vi "Producer consumer.vi"() -> ()   [LabVIEW 2021]
panel:
  in  "stop":bool
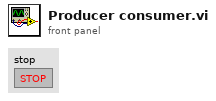
[diagram p1: front panel]
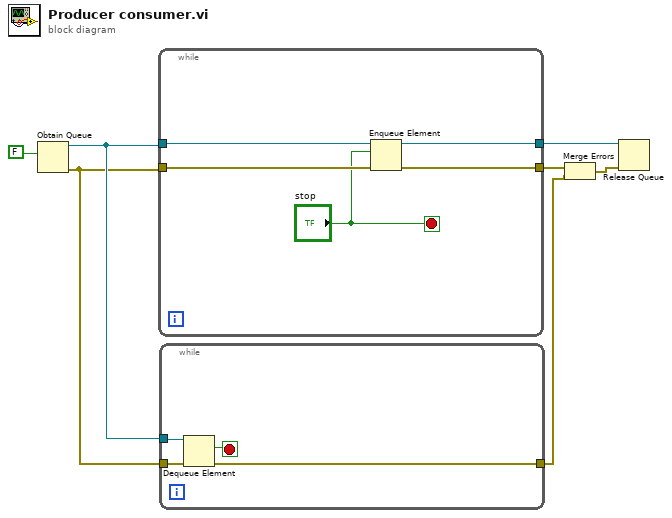
[diagram p0: block diagram]
diagram:
  n1 = Obtain Queue(element data type=FALSE) -> (queue out=w4:refnum<queue>, error out=w3:errorcluster)  [unwired: 4 in, 1 out]
  n2 = while {
    tunnel: w4 -> [w12]
    tunnel: w3 -> [w11]
    tunnel: [w10] -> w7
    tunnel: [w9] -> w6
    stop <- "stop" stop-if-true
    n3 = Enqueue Element(queue=w12, element="stop", error in (no error)=w11) -> (queue out=w10:refnum<queue>, error out=w9:errorcluster)  [unwired: 1 in, 1 out]
  }
  n4 = while {
    tunnel: w4 -> [w16]
    tunnel: w3 -> [w14]
    tunnel: [w13] -> w1
    stop <- w15 stop-if-true
    n5 = Dequeue Element(queue=w16, error in (no error)=w14) -> (element=w15:bool, error out=w13:errorcluster)  [unwired: 1 in, 2 out]
  }
  n6 = Merge Errors(w6, w1) -> (w2:errorcluster)
  n7 = Release Queue(queue=w7, error in (no error)=w2) -> ()  [unwired: 1 in, 3 out]
